vi "Read Status Byte.vi"(7 "Read Status Bit? (F)":bool, 8 "error in (no error)":errorcluster, 9 "Status Bit (Scan Finished)":T1=enum."Scan Finished", 11 "VISA resource name":refnum<visa-resource-name>) -> (0 "error out":errorcluster, 1 "Status Bit":u8, 2 "Status Byte":bool[](array[boolean]), 3 "VISA resource name out":refnum<visa-resource-name>)   [LabVIEW 2015, in "SRS SR400.lvlib"]
doc: "<B>SS { j }</B>\n\nThe SS command reads the status byte. (See the following section for a definition of the status byte). j designates one bit, 0-7, of the status byte. If j is included, the designated bit of the status byte is returned (\"0\" or \"1\"). The bit which is read is then reset. If j is absent, the value of the entire byte is returned (0-255) and all status bits are then reset.\n\nThe definitions for each bit of the status byte are given below:\n\n<B>Bit 0</B>\nParameter Changed from front panel. When this bit is set, it indicates that the front panel knob has been rotated and a setting has been altered.\n\n<B>Bit 1</B>\nData Ready. This bit is set at the end of each count period to indicate that counter data is available.\n\n<B>Bit 2</B>\nScan Finished. This bit is set at the end of a scan if the scan end mode is STOP to indicate that the scan buffer is available for reading. This bit is not set if the scan end mode is START.\n\n<B>Bit 3</B>\nCounter Overrun. This bit is set whenever counter A or B exceeds or equals 10E9 - 1 counts.\n\n<B>Bit 4</B>\nRate Error. This bit is set whenever a gate is missed. This can occur if a gate delay or width exceeds the trigger period minus 1 us.\n\n<B>Bit 5</B>\nRecall Error. This bit is set if a recall from a stored setting detects an error in the recalled data. If an error is found, the instrument setup is not altered.\n\n<B>Bit 6</B>\nSRQ. This bit is always zero when polled via the SS command. This bit is set in the status byte which is read via the GPIB serial poll following a service request generated by the SR400.\n\n<B>Bit 7</B>\nCommand Error. This bit is set when an illegal command is received."
uses:
  SRS SR400.lvlib
  Typedefs/Status Bit.ctl
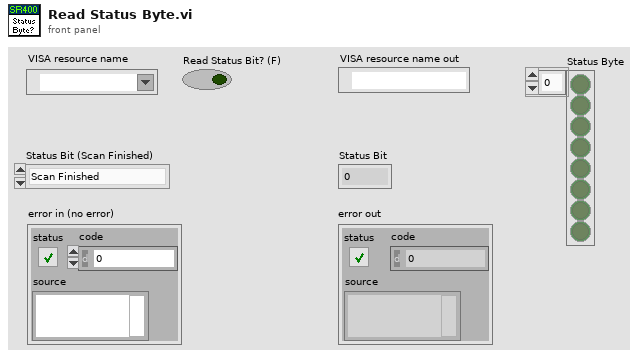
[diagram p1: front panel]
types:
  T1 = typedef "SRS SR400.lvlib/Status Bit.ctl" = enum16{"Parameter Changed", "Data Ready", "Scan Finished", "Counter Overrun", "Rate Error", "Recall Error", "SRQ", "Command Error"}
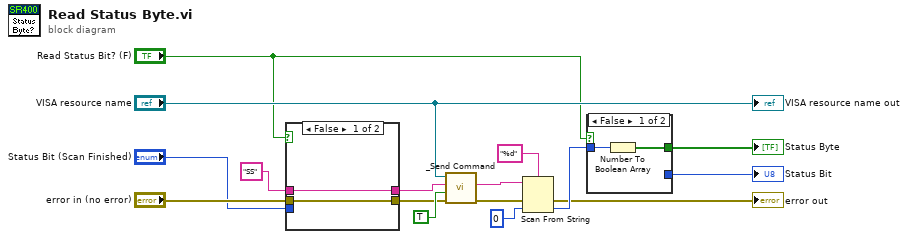
[diagram p0: block diagram]
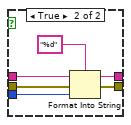
[diagram p3: hidden frame]
diagram:
  n1 = case shown="False" "Read Status Bit? (F)" {
    tunnel: "error in (no error)" -> [w17 w24]
    tunnel: [w17 w23] -> w6
    tunnel: "SS" ("Command") -> [w18 w21]
    tunnel: "Status Bit (Scan Finished)" -> [_ w20]
    tunnel: [w18 w19] -> w3
    frame False {
    }
    frame True {
      n2 = Format Into String(format string="%d", initial string=w21, error in=w24, w20) -> (resulting string=w19:string, error out=w23:errorcluster)
    }
  }
  n3 = call "_Send Command.vi"("error in (no error)"=w6, "Read Value? (F)"=TRUE ("Query? (F)"), "Command"=w3, "VISA resource name"="VISA resource name") -> ("error out"=w10:errorcluster, "Response"=w11:string)  [unwired: 5 in, 1 out]
  n4 = Scan From String(format string="%d", input string=w11, error in=w10, default 1=u8 0 ("default value 1")) -> (error out=→"error out":errorcluster, output 1=w12:u8)  [unwired: 1 in, 2 out]
  n5 = case shown="False" "Read Status Bit? (F)" {
    tunnel: [w26 _] -> w15
    tunnel: w12 -> [w25 w27]
    tunnel: [_ w27] -> w1
    frame False {
      n6 = Number To Boolean Array(number=w25) -> (Boolean array=w26:bool[])
    }
    frame True {
    }
  }
  "Status Byte" <- w15
  "Status Bit" <- w1
  "VISA resource name out" <- "VISA resource name"
